vi "AddControlsToControlStateArray.vi"(8 "error in (no error)":errorcluster, 10 "Array":refnum<vi>[](array[refnum]), 11 "Control State Array":T1[](array[typedef])) -> (0 "error out":errorcluster, 3 "Control State Array (out)":T1[](array[typedef]))   [LabVIEW 2010]
doc: "Adds new control references to array of control states. States are: Visible (T/F), Enabled (Enabled, Disabled, Disabled and greyed out)"
uses:
  Types/ControlAttributes.ctl
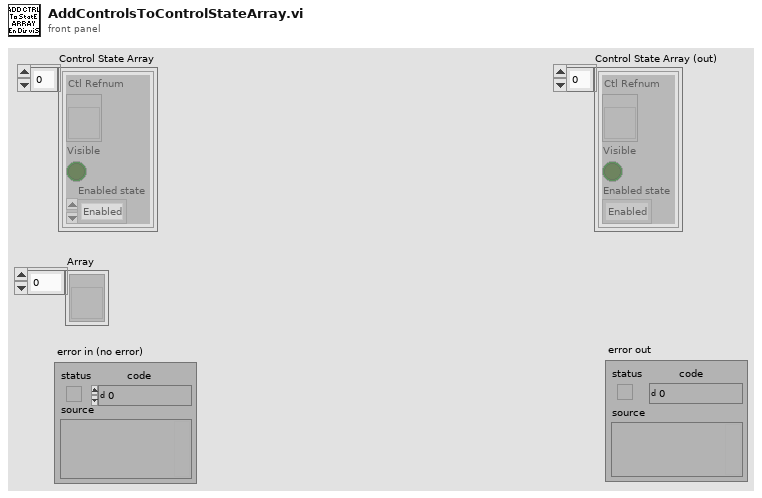
[diagram p1: front panel]
types:
  T1 = typedef "ControlAttributes.ctl" = cluster{"Ctl Refnum":refnum<vi>, "Visible":bool, "Enabled state":enum8{"Enabled", "Disabled", "Disabled and Grayed Out"}}
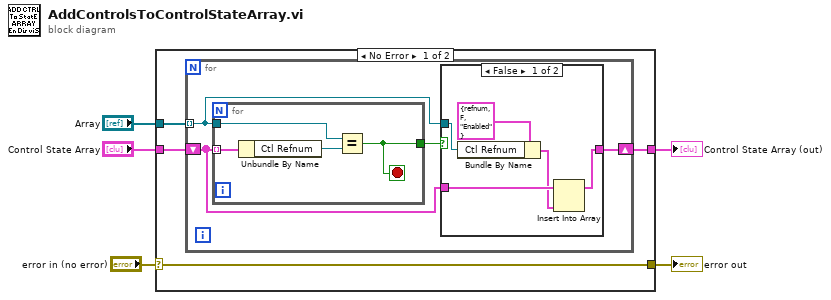
[diagram p0: block diagram]
diagram:
  n1 = case shown="No Error" "error in (no error)" {
    selector: "error in (no error)" -> [w9 w25]
    tunnel: [w9 w25] -> w4
    tunnel: "Control State Array" -> [w7 w24]
    tunnel: "Array" -> [w6 _]
    tunnel: [w8 w24] -> w1
    frame No Error {
      n2 = for {
        tunnel: w6 -> [w10] mode=indexing
        shift-right: [w13] -> w8
        shift-left: w7 -> [w12]
        n3 = for {
          tunnel: w12 -> [w22] mode=indexing
          tunnel: w10 -> [w20]
          tunnel: [w21] -> w11
          stop <- w21 stop-if-true
          n4 = Unbundle By Name(w22) -> ("Ctl Refnum"=w23:refnum<vi>)
          n5 = Equal?(x=w20, y=w23) -> (x = y?=w21:bool)
        }
        n6 = case shown="False" w11 {
          tunnel: [w18 w19] -> w13
          tunnel: w12 -> [w17 w19]
          tunnel: w10 -> [w14 _]
          frame False {
            n7 = Bundle By Name(cluster=T1 {"Ctl Refnum"=refnum, "Visible"=FALSE, "Enabled state"=enum."Enabled"} ("Control Attributes"), "Ctl Refnum"=w14) -> (w15:T1)
            n8 = Insert Into Array(array=w17, new element=w15) -> (w18:T1[])  [unwired: 1 in]
          }
          frame True {
          }
        }
      }
    }
    frame Error {
    }
  }
  "error out" <- w4
  "Control State Array (out)" <- w1
